vi "Parse-broadcast-data-system.vi"(8 "error in (no error)":errorcluster, 10 "Multiple device identification XML string":string="<LecList>\n  <Lec name='EC_Alpha' ip='192.168.42.30' mac='address' />\n  <Lec name='EC_Beta' ip='192.168.42.31' mac='addressB' />\n</LecList>") -> (0 "error out":errorcluster, 2 "System information":T1)   [LabVIEW 2013, in "MaterialCharacterization.lvlib" / "MC-SM1000.lvclass"]
uses:
  MC-SM1000.lvclass
  System-information.ctl
  <vilib>/xml/Load XML String.vi
  <vilib>/xml/Close Reference(Node).vi
  <vilib>/xml/NI_XML.lvlib
  <resource>/objmgr/DOMUserDefRef.rc
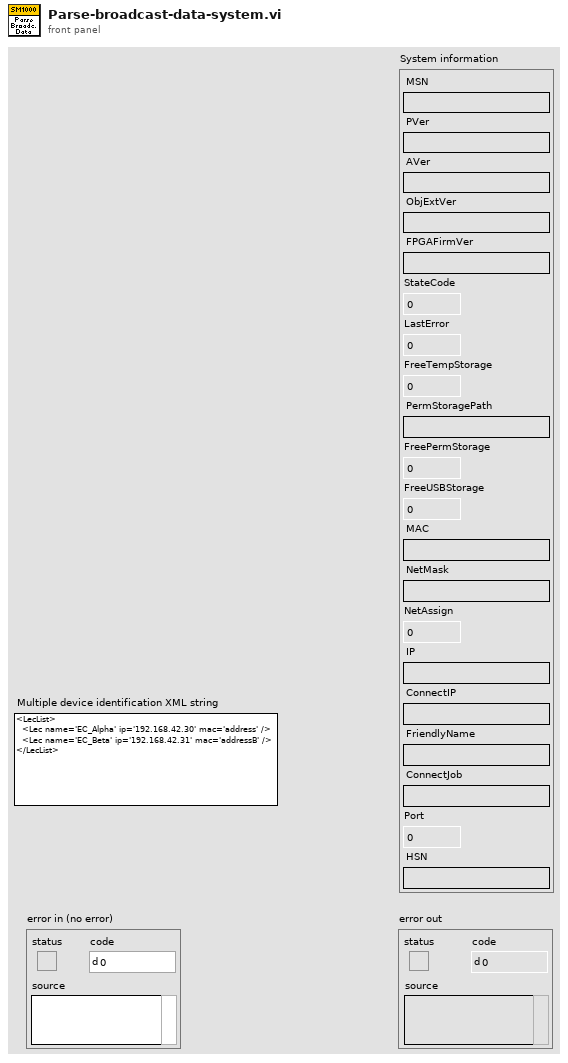
[diagram p1: front panel]
types:
  T1 = typedef "MaterialCharacterization.lvlib/MC-SM1000.lvclass/System-information.ctl" = cluster{"MSN":string, "PVer":string, "AVer":string, "ObjExtVer":string, "FPGAFirmVer":string, "StateCode":u32, "LastError":i32, "FreeTempStorage":u32, "PermStoragePath":string, "FreePermStorage":u32, "FreeUSBStorage":u32, "MAC":string, "NetMask":string, "NetAssign":i32, "IP":string, "ConnectIP":string, "FriendlyName":string, "ConnectJob":string, "Port":u32, "HSN":string}
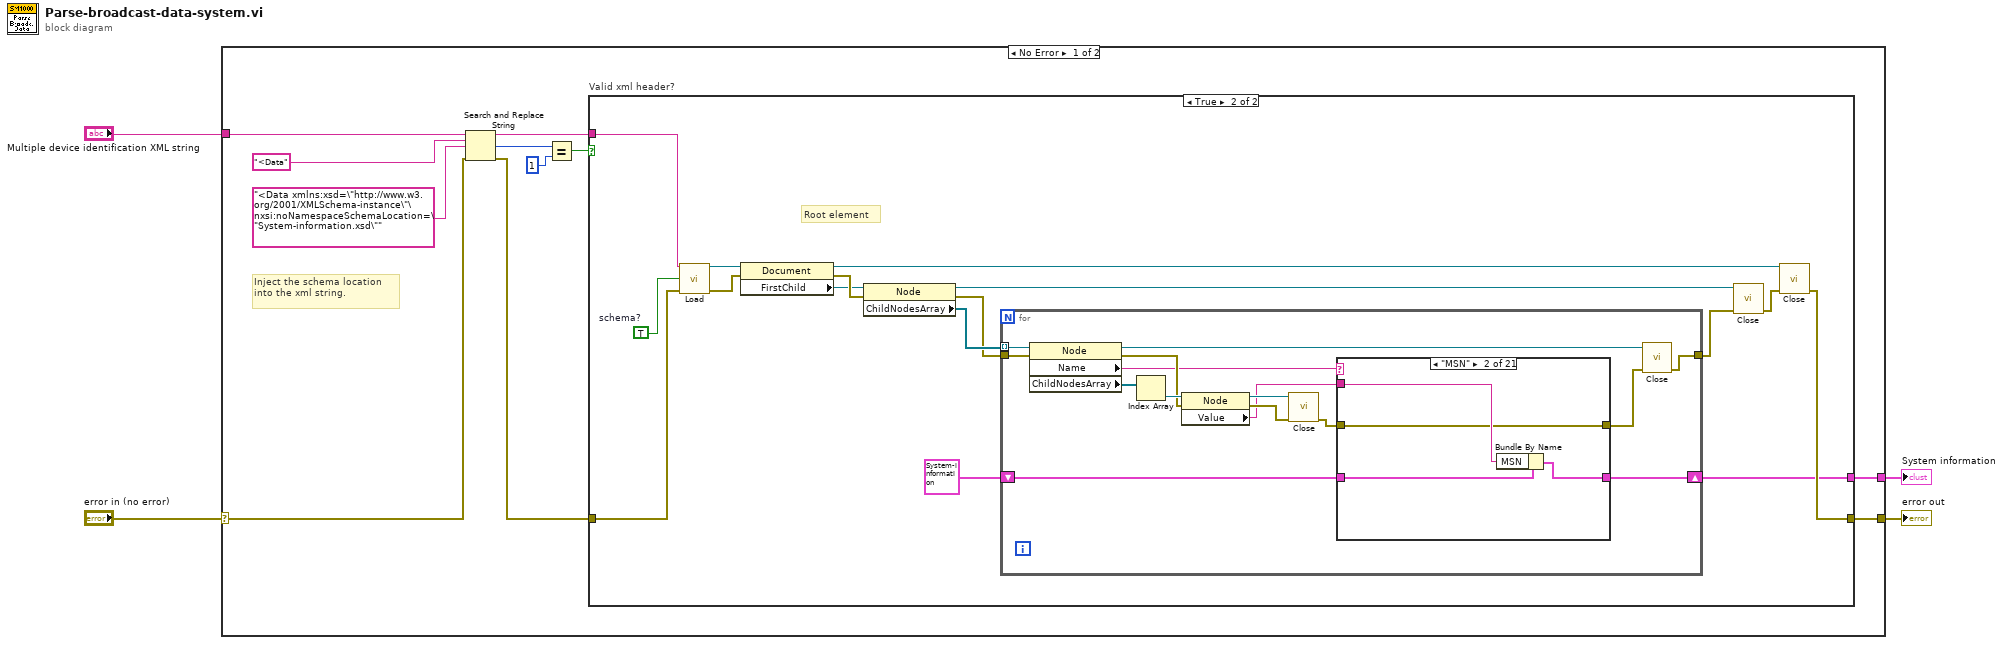
[diagram p0: block diagram]
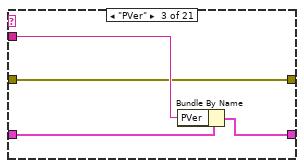
[diagram p4: hidden frame]
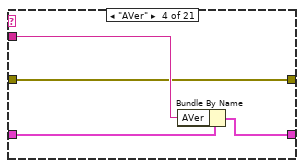
[diagram p5: hidden frame]
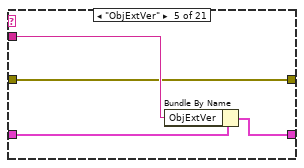
[diagram p6: hidden frame]
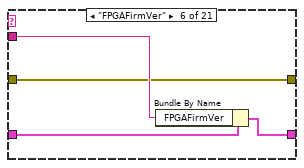
[diagram p7: hidden frame]
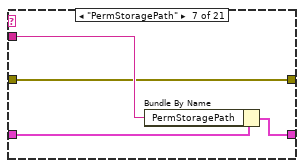
[diagram p8: hidden frame]
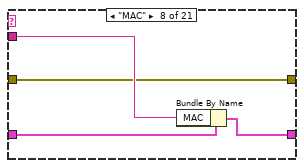
[diagram p9: hidden frame]
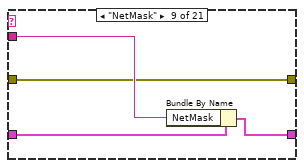
[diagram p10: hidden frame]
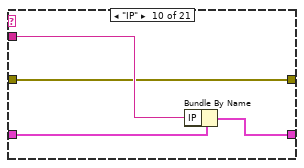
[diagram p11: hidden frame]
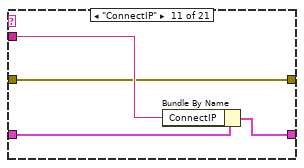
[diagram p12: hidden frame]
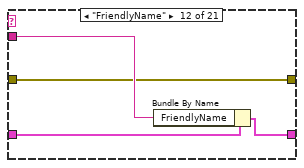
[diagram p13: hidden frame]
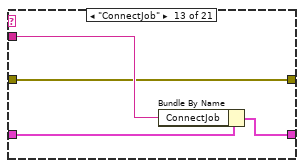
[diagram p14: hidden frame]
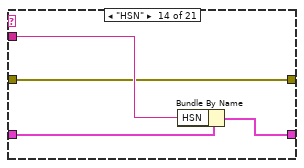
[diagram p15: hidden frame]
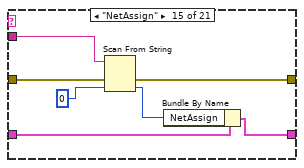
[diagram p16: hidden frame]
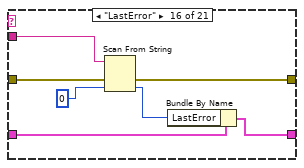
[diagram p17: hidden frame]
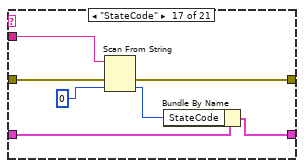
[diagram p18: hidden frame]
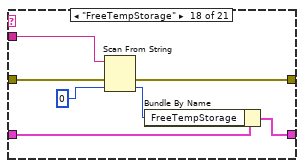
[diagram p19: hidden frame]
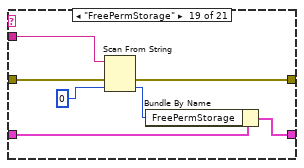
[diagram p20: hidden frame]
diagram:
  n1 = case shown="No Error" "error in (no error)" {
    selector: "error in (no error)" -> [w12 w151]
    tunnel: [w7 w151] -> w3
    tunnel: "Multiple device identification XML string" -> [w15 _]
    tunnel: [w5 _] -> w1
    frame No Error {
      # "Inject the schema location\ninto the xml string."
      n2 = Search and Replace String(input string=w15, search string="<Data", replace string="<Data xmlns:xsd=\"http://www.w3.org/2001/XMLSchema-instance\"\nxsi:noNamespaceSchemaLocation=\"System-information.xsd\"", error in=w12) -> (result string=w8:string, number of replacements=w11:i32, error out=w6:errorcluster)  [unwired: 4 in, 1 out]
      n3 = Equal?(x=w11, y=1) -> (x = y?=w9:bool)
      n4 = case "Valid xml header?" shown="True" w9 {
        tunnel: w8 -> [_ w19]
        tunnel: [w16 w28] -> w7
        tunnel: w6 -> [w16 w29]
        tunnel: [_ w17] -> w5
        frame False {
        }
        frame True {
          w32 = TRUE  # schema?
          # "Root element"
          n5 = call-poly <vilib>:"Load.vi"("XML string"=w19, "process schema (False)"=w32, "error in (no error)"=w29) -> ("DOM document out"=w31:refnum<k20>, "error out"=w30:errorcluster)  [unwired: 10 in, 1 out]
          n6 = property class="Document"(reference=w31, error in=w30) -> (reference out=w21:refnum<k20>, error out=w23:errorcluster, "FirstChild"=w20:refnum<k20>)
          n7 = property class="Node"(reference=w20, error in=w23) -> (reference out=w22:refnum<k20>, error out=w24:errorcluster, "ChildNodesArray"=w25:refnum<k20>[])
          n8 = for {
            tunnel: w25 -> [w38] mode=indexing
            tunnel: w24 -> [w37]
            tunnel: [w46] -> w27
            shift-right: [w44] -> w17
            shift-left: T1 {"MSN"="", "PVer"="", "AVer"="", "ObjExtVer"="", "FPGAFirmVer"="", "StateCode"=0, "LastError"=0, "FreeTempStorage"=0, "PermStoragePath"="", "FreePermStorage"=0, "FreeUSBStorage"=0, "MAC"="", "NetMask"="", "NetAssign"=0, "IP"="", "ConnectIP"="", "FriendlyName"="", "ConnectJob"="", "Port"=0, "HSN"=""} ("System information") -> [w45]
            n9 = property class="Node"(reference=w38, error in=w37) -> (reference out=w36:refnum<k20>, error out=w41:errorcluster, "Name"=w35:string, "ChildNodesArray"=w43:refnum<k20>[])
            n10 = Index Array(array=w43) -> (element=w42:refnum<k20>)  [unwired: 1 in]
            n11 = property class="Node"(reference=w42, error in=w41) -> (reference out=w39:refnum<k20>, error out=w40:errorcluster, "Value"=w33:string)
            n12 = call-poly <vilib>:"Close.vi"("error in (no error)"=w40, "node"=w39) -> ("error out"=w34:errorcluster)  [unwired: 7 in]
            n13 = case shown="\"MSN\"" w35 {
              tunnel: w34 -> [w49 w50 w54 w58 w62 w66 w70 w74 w78 w82 w86 w90 w94 w98 w106 w113 w120 w127 w134 w141 w148]
              tunnel: [w49 w50 w54 w58 w62 w66 w70 w74 w78 w82 w86 w90 w94 w98 w102 w109 w116 w123 w130 w137 w144] -> w47
              tunnel: w45 -> [w48 w53 w57 w61 w65 w69 w73 w77 w81 w85 w89 w93 w97 w101 w108 w115 w122 w129 w136 w143 w150]
              tunnel: w33 -> [_ w51 w55 w59 w63 w67 w71 w75 w79 w83 w87 w91 w95 w99 w105 w112 w119 w126 w133 w140 w147]
              tunnel: [w48 w52 w56 w60 w64 w68 w72 w76 w80 w84 w88 w92 w96 w100 w107 w114 w121 w128 w135 w142 w149] -> w44
              frame Default {
              }
              frame "MSN" {
                n14 = Bundle By Name(cluster=w53, "MSN"=w51) -> (w52:T1)
              }
              frame "PVer" {
                n15 = Bundle By Name(cluster=w57, "PVer"=w55) -> (w56:T1)
              }
              frame "AVer" {
                n16 = Bundle By Name(cluster=w61, "AVer"=w59) -> (w60:T1)
              }
              frame "ObjExtVer" {
                n17 = Bundle By Name(cluster=w65, "ObjExtVer"=w63) -> (w64:T1)
              }
              frame "FPGAFirmVer" {
                n18 = Bundle By Name(cluster=w69, "FPGAFirmVer"=w67) -> (w68:T1)
              }
              frame "PermStoragePath" {
                n19 = Bundle By Name(cluster=w73, "PermStoragePath"=w71) -> (w72:T1)
              }
              frame "MAC" {
                n20 = Bundle By Name(cluster=w77, "MAC"=w75) -> (w76:T1)
              }
              frame "NetMask" {
                n21 = Bundle By Name(cluster=w81, "NetMask"=w79) -> (w80:T1)
              }
              frame "IP" {
                n22 = Bundle By Name(cluster=w85, "IP"=w83) -> (w84:T1)
              }
              frame "ConnectIP" {
                n23 = Bundle By Name(cluster=w89, "ConnectIP"=w87) -> (w88:T1)
              }
              frame "FriendlyName" {
                n24 = Bundle By Name(cluster=w93, "FriendlyName"=w91) -> (w92:T1)
              }
              frame "ConnectJob" {
                n25 = Bundle By Name(cluster=w97, "ConnectJob"=w95) -> (w96:T1)
              }
              frame "HSN" {
                n26 = Bundle By Name(cluster=w101, "HSN"=w99) -> (w100:T1)
              }
              frame "NetAssign" {
                n27 = Scan From String(input string=w105, error in=w106, default 1=0) -> (error out=w102:errorcluster, output 1=w103:i32)  [unwired: 2 in, 2 out]
                n28 = Bundle By Name(cluster=w108, "NetAssign"=w103) -> (w107:T1)
              }
              frame "LastError" {
                n29 = Scan From String(input string=w112, error in=w113, default 1=0) -> (error out=w109:errorcluster, output 1=w110:i32)  [unwired: 2 in, 2 out]
                n30 = Bundle By Name(cluster=w115, "LastError"=w110) -> (w114:T1)
              }
              frame "StateCode" {
                n31 = Scan From String(input string=w119, error in=w120, default 1=u32 0) -> (error out=w116:errorcluster, output 1=w117:u32)  [unwired: 2 in, 2 out]
                n32 = Bundle By Name(cluster=w122, "StateCode"=w117) -> (w121:T1)
              }
              frame "FreeTempStorage" {
                n33 = Scan From String(input string=w126, error in=w127, default 1=u32 0) -> (error out=w123:errorcluster, output 1=w124:u32)  [unwired: 2 in, 2 out]
                n34 = Bundle By Name(cluster=w129, "FreeTempStorage"=w124) -> (w128:T1)
              }
              frame "FreePermStorage" {
                n35 = Scan From String(input string=w133, error in=w134, default 1=u32 0) -> (error out=w130:errorcluster, output 1=w131:u32)  [unwired: 2 in, 2 out]
                n36 = Bundle By Name(cluster=w136, "FreePermStorage"=w131) -> (w135:T1)
              }
              frame "FreeUSBStorage" {
                n37 = Scan From String(input string=w140, error in=w141, default 1=u32 0) -> (error out=w137:errorcluster, output 1=w138:u32)  [unwired: 2 in, 2 out]
                n38 = Bundle By Name(cluster=w143, "FreeUSBStorage"=w138) -> (w142:T1)
              }
              frame "Port" {
                n39 = Scan From String(input string=w147, error in=w148, default 1=u32 0) -> (error out=w144:errorcluster, output 1=w145:u32)  [unwired: 2 in, 2 out]
                n40 = Bundle By Name(cluster=w150, "Port"=w145) -> (w149:T1)
              }
            }
            n41 = call-poly <vilib>:"Close.vi"("error in (no error)"=w47, "node"=w36) -> ("error out"=w46:errorcluster)  [unwired: 7 in]
          }
          n42 = call-poly <vilib>:"Close.vi"("error in (no error)"=w27, "node"=w22) -> ("error out"=w26:errorcluster)  [unwired: 7 in]
          n43 = call-poly <vilib>:"Close.vi"("error in (no error)"=w26, "node"=w21) -> ("error out"=w28:errorcluster)  [unwired: 7 in]
        }
      }
    }
    frame Error {
    }
  }
  "error out" <- w3
  "System information" <- w1
